vi "soundstudio.vi"() -> ()   [LabVIEW 2017]
uses:
  <vilib>/sound2/lvsound2.llb/Sound Data Format.ctl
  <vilib>/sound2/lvsound2.llb/Sampling Mode.ctl
  <vilib>/Analysis/3filter.llb/Filter Passband Type.ctl
  <vilib>/Analysis/3filter.llb/Savitzky-Golay Filter (DBL).vi
  <vilib>/sound2/lvsound2.llb/Sound File Info (path).vi
  <vilib>/sound2/lvsound2.llb/Sound File Write Open.vi
  <vilib>/sound2/lvsound2.llb/Sound Input Read (DBL).vi
  <vilib>/sound2/lvsound2.llb/Sound File Write (DBL).vi
  <vilib>/Analysis/3filter.llb/Butterworth Filter (DBL).vi
  <vilib>/Waveform/WDTOps.llb/WDT Number of Waveform Samples DBL.vi
  <vilib>/Analysis/NI_AALBase.lvlib
panel:
  in  "Noise":dbl(slide) scale=0.0..10.0
  in  "Smooth":i32(slide)=2 scale=2.0..10.0
  in  "Filter cutoff (Hz)":dbl(slide)=1557.5757575757575 scale=50.0..5000.0
  in  "Filter":enum16{"None", "Low pass", "High pass"}(ring)
  in  "Reverse":enum32{"Radio Selection 1", "Radio Selection 2"}(radio)=enum."Radio Selection 2"
  in  "Speed":dbl(slide)=1.0 scale=0.5..2.0
  in  "Test effects":bool
  in  "Cancel":bool
  in  "Apply":bool
  in  "Record settings":T1={"sample rate (S/s)"=22050.0, "number of channels"=2, "bits per sample"=16}
  in  "Record":bool
  in  "Stop":bool
  in  "Play":bool
  in  "Stop program":bool
  in  "Load audio":bool
  in  "Save audio as":path=path "C:/Users/Yugo/Downloads/modified.wav"
  in  "Save audio":bool
  out "Waveform Graph":waveform(dbl)[](graph)=[{"t0"=timestamp(0 s since 1904-01-01), "dt"=2.2675736961451248e-05, "Y"=array[77948 elements]}]
  in  "Load file:":path=path "C:/Users/Yugo/Downloads/AintNobody.wav"
  # "EFFECTS"
  # "OR"
  # "Play"
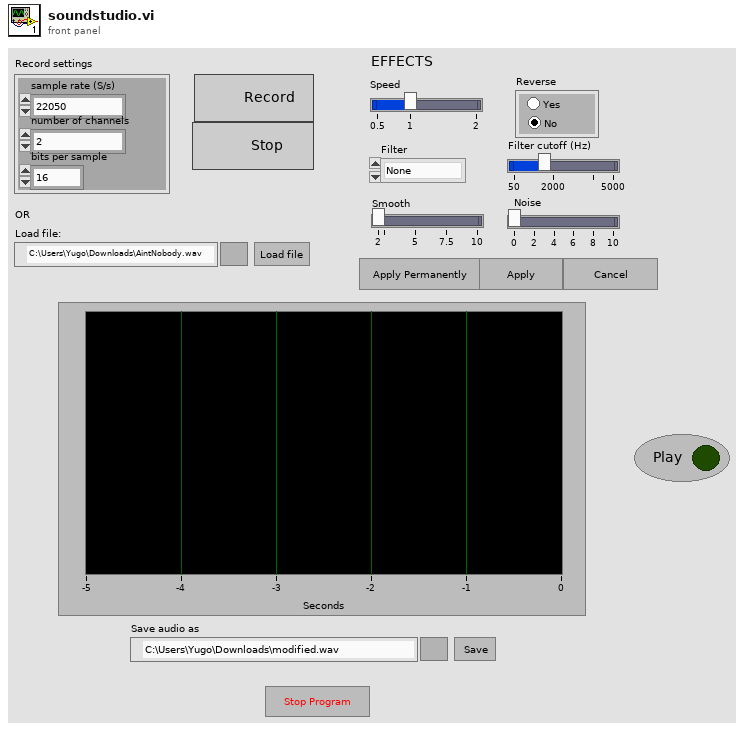
[diagram p1: front panel]
types:
  T1 = typedef "Sound Data Format.ctl" = cluster{"sample rate (S/s)":dbl, "number of channels":i32, "bits per sample":i32}
  T2 = typedef "NI_AALBase.lvlib/Filter Passband Type.ctl" = enum32{"Lowpass", "Highpass", "Bandpass", "Bandstop"}
  T3 = typedef "Sampling Mode.ctl" = i32
  T4 = typedef "Sound File Refnum.ctl" = refnum<file>
  T5 = typedef "Sound Input Task ID.ctl" = u32
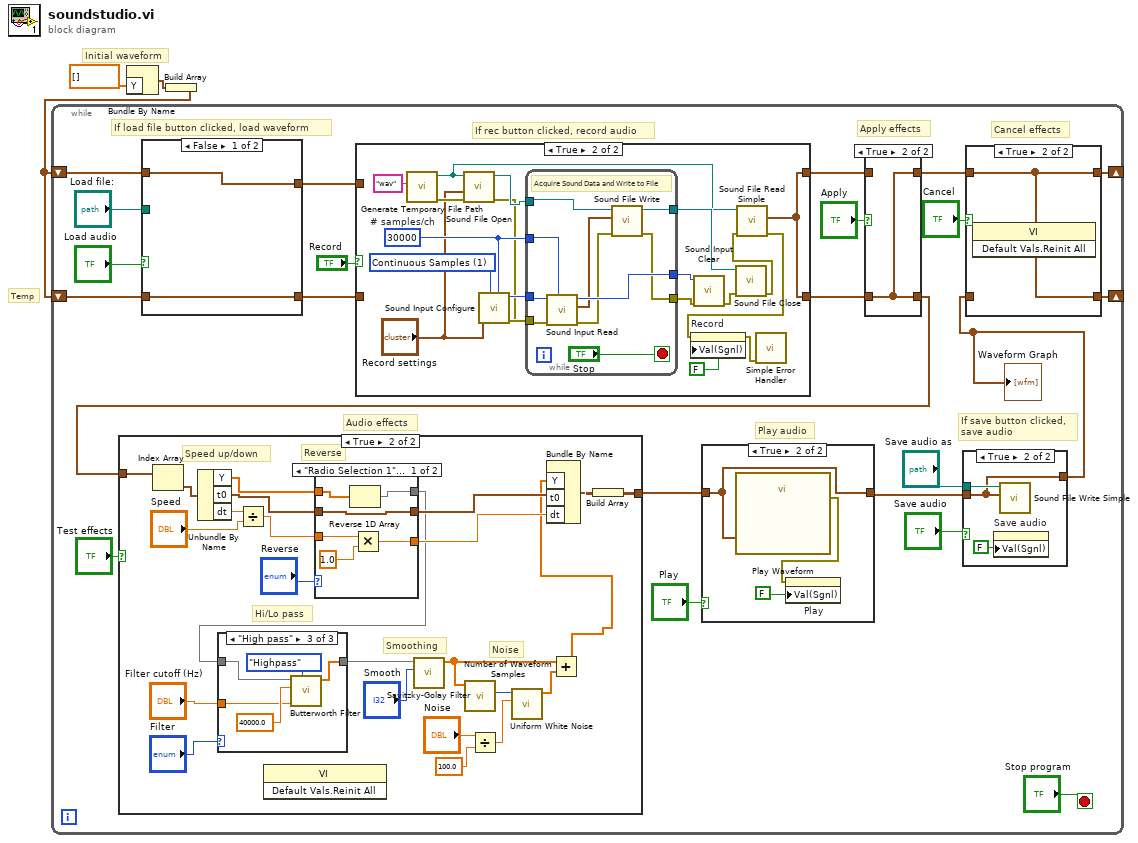
[diagram p0: block diagram]
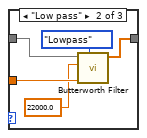
[diagram p4: hidden frame]
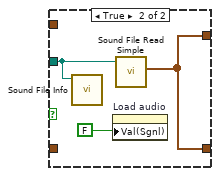
[diagram p10: hidden frame]
diagram:
  # "Temp"
  # "Initial waveform"
  n1 = Bundle By Name("Y"=dbl[] []) -> (w3:waveform(dbl))  [unwired: 1 in]
  n2 = Build Array(w3) -> (w1:waveform(dbl)[])
  n3 = while {
    shift-right: [w9] -> _
    shift-left: w1 -> [w21]
    shift-right: [w10] -> _
    shift-left: w1 -> [w16]
    stop <- "Stop program" stop-if-true
    # "Audio effects"
    # "Cancel effects"
    # "Play audio"
    # "Apply effects"
    # "If rec button clicked, record audio"
    # "If save button clicked, \nsave audio"
    # "If load file button clicked, load waveform"
    n4 = case shown="False" "Load audio" {
      tunnel: "Load file:" -> [_ w117]
      tunnel: w21 -> [w114 _]
      tunnel: [w114 w115] -> w20
      tunnel: w16 -> [w113 _]
      tunnel: [w113 w115] -> w15
      frame False {
      }
      frame True {
        n5 = call-poly <vilib>:"Sound File Info.vi"("path"=w117) -> ()  [unwired: 7 in, 4 out]
        n6 = property on="Load audio" class="Bool (strict)"("Val(Sgnl)"=FALSE) -> ()  [unwired: 2 in, 2 out]
        n7 = call <vilib>:"Sound File Read Simple.vi"("path"=w117) -> ("data"=w115:waveform(dbl)[])  [unwired: 7 in, 3 out]
      }
    }
    n8 = case shown="True" "Record" {
      tunnel: w20 -> [w83 _]
      tunnel: [w83 w84] -> w13
      tunnel: w15 -> [w82 _]
      tunnel: [w82 w84] -> w6
      frame False {
      }
      frame True {
        w98 = 30000  # # samples/ch
        w97 = T3 1 items=["Finite Samples", "Continuous Samples"] ("sample mode")
        n9 = call <vilib>:"Generate Temporary File Path.vi"("Temporary File Extension (tmp)"="wav") -> ("error out"=w92:errorcluster, "Unique Temporary File Path"=w89:path)  [unwired: 9 in]
        n10 = call-poly <vilib>:"Sound File Open.vi"("error in (no error)"=w92, "sound format"="Record settings", "path"=w89) -> ("error out"=w93:errorcluster, "sound file refnum"=w96:T4)  [unwired: 7 in]
        n11 = call <vilib>:"Sound Input Configure.vi"("number of samples/ch"=w98, "sample mode"=w97, "error in (no error)"=w93, "sound format"="Record settings") -> ("error out"=w102:errorcluster, "task ID"=w101:T5)  [unwired: 6 in]
        n12 = while {
          tunnel: w98 -> [w109]
          tunnel: w96 -> [w108]
          tunnel: [w107] -> w95
          tunnel: w101 -> [w111]
          tunnel: [w110] -> w100
          tunnel: w102 -> [w112]
          tunnel: [w104] -> w99
          stop <- "Stop" stop-if-true
          # "Acquire Sound Data and Write to File"
          n13 = call-poly <vilib>:"Sound Input Read.vi"("number of samples/ch"=w109, "error in (no error)"=w112, "task ID"=w111) -> ("error out"=w106:errorcluster, "data"=w105:waveform(dbl)[], "task ID out"=w110:T5)  [unwired: 6 in]
          n14 = call-poly <vilib>:"Sound File Write.vi"("error in (no error)"=w106, "data"=w105, "sound file refnum"=w108) -> ("error out"=w104:errorcluster, "sound file refnum out"=w107:T4)  [unwired: 7 in]
        }
        n15 = call <vilib>:"Sound Input Clear.vi"("error in (no error)"=w99, "task ID"=w100) -> ("error out"=w94:errorcluster)  [unwired: 9 in]
        n16 = call <vilib>:"Sound File Close.vi"("error in (no error)"=w94, "sound file refnum"=w95) -> ("error out"=w90:errorcluster)  [unwired: 9 in]
        n17 = call <vilib>:"Sound File Read Simple.vi"("error in (no error)"=w90, "path"=w89) -> ("error out"=w87:errorcluster, "data"=w84:waveform(dbl)[])  [unwired: 6 in, 2 out]
        n18 = property on="Record" class="Bool (strict)"(error in=w87, "Val(Sgnl)"=FALSE) -> (error out=w88:errorcluster)  [unwired: 1 in, 1 out]
        n19 = call <vilib>:"Simple Error Handler.vi"("error in (no error)"=w88) -> ()  [unwired: 4 in, 5 out]
      }
    }
    n20 = case shown="True" "Apply" {
      tunnel: w13 -> [w76 _]
      tunnel: [w76 w77] -> w11
      tunnel: w6 -> [w75 w77]
      tunnel: [w75 w77] -> w4
      frame False {
      }
      frame True {
      }
    }
    n21 = case shown="True" "Test effects" {
      tunnel: w4 -> [w27 w51]
      tunnel: [w27 w45] -> w8
      frame False {
      }
      frame True {
        # "Noise"
        # "Smoothing"
        # "Hi/Lo pass"
        # "Reverse"
        # "Speed up/down"
        n22 = Index Array(array=w51) -> (element=w50:waveform(dbl))  [unwired: 1 in]
        n23 = Unbundle By Name(w50) -> ("Y"=w42:dbl[], "t0"=w41:timestamp, "dt"=w48:dbl)
        n24 = Divide(x=w48, y="Speed") -> (x/y=w44:dbl)
        n25 = invoke class="VI" method="Default Vals.Reinit All"() -> ()  [unwired: 3 in, 3 out]
        n26 = case shown="\"Radio Selection 1\", Default" "Reverse" {
          tunnel: w44 -> [w68 w71]
          tunnel: [w66 w71] -> w43
          tunnel: w42 -> [w65 w70]
          tunnel: w41 -> [w64 w69]
          tunnel: [w63 w70] -> w38
          tunnel: [w64 w69] -> w40
          frame "Radio Selection 1", Default {
            n27 = Reverse 1D Array(array=w65) -> (reversed array=w63:dbl[])
            n28 = Multiply(x=w68, y=1.0) -> (x*y=w66:dbl)
          }
          frame "Radio Selection 2" {
          }
        }
        n29 = case shown="\"High pass\"" "Filter" {
          tunnel: w38 -> [w52 w56 w62]
          tunnel: [w52 w55 w61] -> w36
          tunnel: "Filter cutoff (Hz)" -> [_ w57 w58]
          frame "None", Default {
          }
          frame "Low pass" {
            n30 = call-poly <vilib>:"Butterworth Filter.vi"("filter type"=Filter_Passband_Type."Lowpass", "low cutoff freq: fl"=w57, "sampling freq: fs"=22000.0, "X"=w56) -> ("Filtered X"=w55:dbl[])  [unwired: 4 in, 1 out]
          }
          frame "High pass" {
            n31 = call-poly <vilib>:"Butterworth Filter.vi"("filter type"=Filter_Passband_Type."Highpass", "low cutoff freq: fl"=w58, "sampling freq: fs"=40000.0, "X"=w62) -> ("Filtered X"=w61:dbl[])  [unwired: 4 in, 1 out]
          }
        }
        n32 = call-poly <vilib>:"Savitzky-Golay Filter.vi"("side points"="Smooth", "X"=w36) -> ("Filtered X"=w33:dbl[])  [unwired: 8 in, 1 out]
        n33 = call-poly <vilib>:"Number of Waveform Samples.vi"("waveform in"=w33) -> ("number of samples"=w29:i32)  [unwired: 8 in, 2 out]
        n34 = Divide(x="Noise", y=100.0) -> (x/y=w32:dbl)
        n35 = call <vilib>:"Uniform White Noise.vi"("amplitude"=w32, "samples"=w29) -> ("uniform white noise"=w34:dbl[])  [unwired: 8 in, 1 out]
        n36 = Add(x=w33, y=w34) -> (x+y=w28:dbl[])
        n37 = Bundle By Name("Y"=w28, "t0"=w40, "dt"=w43) -> (w46:waveform(dbl))  [unwired: 1 in]
        n38 = Build Array(w46) -> (w45:waveform(dbl)[])
      }
    }
    n39 = case shown="True" "Play" {
      tunnel: w8 -> [w78 w80]
      tunnel: [w78 w80] -> w18
      frame False {
      }
      frame True {
        n40 = call "Play Waveform"("Data"=w80) -> ("error out"=w79:errorcluster)  [unwired: 18 in]
        n41 = property on="Play" class="Bool (strict)"(error in=w79, "Val(Sgnl)"=FALSE) -> ()  [unwired: 1 in, 2 out]
      }
    }
    n42 = case shown="True" "Save audio" {
      tunnel: w18 -> [w118 w119]
      tunnel: "Save audio as" -> [_ w121]
      tunnel: [w118 w119] -> w5
      frame False {
      }
      frame True {
        n43 = property on="Save audio" class="Bool (strict)"("Val(Sgnl)"=FALSE) -> ()  [unwired: 2 in, 2 out]
        n44 = call <vilib>:"Sound File Write Simple.vi"("data"=w119, "path"=w121) -> ()  [unwired: 8 in, 2 out]
      }
    }
    "Waveform Graph" <- w5
    n45 = case shown="True" "Cancel" {
      tunnel: w11 -> [w73 w74]
      tunnel: w5 -> [w72 _]
      tunnel: [w73 w74] -> w9
      tunnel: [w72 w74] -> w10
      frame False {
      }
      frame True {
        n46 = invoke class="VI" method="Default Vals.Reinit All"() -> ()  [unwired: 3 in, 3 out]
      }
    }
  }
